vi "TGI_.vi"(1 "Signals":dbl[](array[numeric]), 2 "Hadamard":bool[][](array[boolean]), 3 "Initialise Array":dbl[](array[numeric])) -> (0 "Reconstruction":dbl[](array[numeric]))   [LabVIEW 2020]
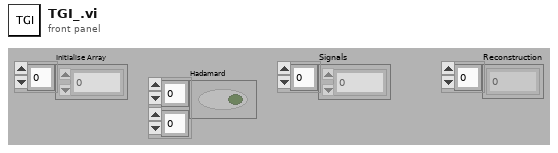
[diagram p1: front panel]
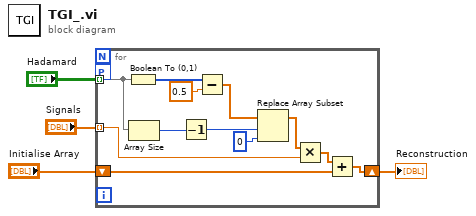
[diagram p0: block diagram]
diagram:
  n1 = for {
    tunnel: "Signals" -> [w15] mode=indexing
    tunnel: "Hadamard" -> [w16] mode=indexing
    shift-right: [w14] -> w4
    shift-left: "Initialise Array" -> [w13]
    workers-P: _ -> [_]
    n2 = Boolean To (0,1)(Boolean=w16) -> (0, 1=w12:i16[])
    n3 = Array Size(array=w16) -> (size(s)=w5:i32)
    n4 = Decrement(x=w5) -> (x-1=w6:i32)
    n5 = Subtract(x=w12, y=0.5) -> (x-y=w9:dbl[])
    n6 = Replace Array Subset(array=w9, new element=0 ("index"), index=w6) -> (w7:dbl[])
    n7 = Multiply(x=w7, y=w15) -> (x*y=w10:dbl[])
    n8 = Add(x=w10, y=w13) -> (x+y=w14:dbl[])
  }
  "Reconstruction" <- w4
